vi "UsingCaseStructures.vi"() -> ()   [LabVIEW 2018]
panel:
  in  "Numeric":i32
  in  "stop":bool
  in  "Temperature":dbl(slide) scale=0.0..200.0
  out "Thermometer":dbl(slide) scale=0.0..100.0
  in  "milliseconds to wait":i32=100
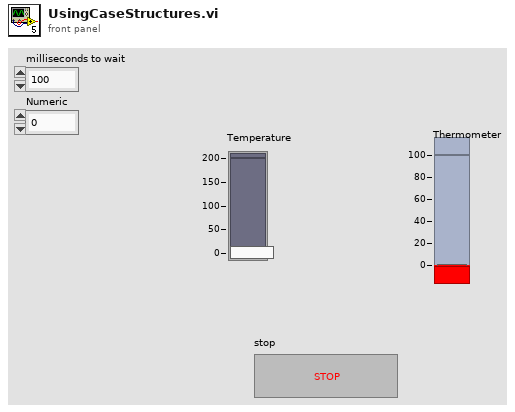
[diagram p1: front panel]
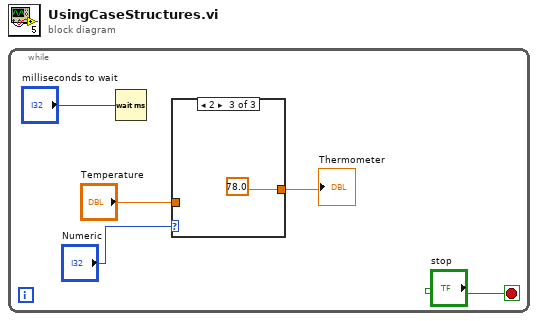
[diagram p0: block diagram]
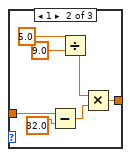
[diagram p3: hidden frame]
diagram:
  n1 = while {
    stop <- "stop" stop-if-true
    n2 = Wait (ms)(milliseconds to wait="milliseconds to wait") -> ()  [unwired: 1 out]
    n3 = case shown="2" "Numeric" {
      tunnel: "Temperature" -> [w6 w13 _]
      tunnel: [w6 w11 78.0 ("Numeric 2")] -> w2
      frame 0, Default {
      }
      frame 1 {
        n4 = Subtract(x=w13, y=32.0) -> (x-y=w12:dbl)
        n5 = Divide(x=5.0, y=9.0) -> (x/y=w10:dbl)
        n6 = Multiply(x=w10, y=w12) -> (x*y=w11:dbl)
      }
      frame 2 {
      }
    }
    "Thermometer" <- w2
  }
